vi "Duplicate.vi"(8 "error in":errorcluster, 10 "parameters":variant, 11 "node in":refnum<class "module editor node.lvclass">) -> (0 "error out":errorcluster, 3 "node copy out":refnum<class "module editor node.lvclass">)   [LabVIEW 2013, in "PL Framework Configuration Tool.lvlib" / "module editor node.lvclass"]
doc: "Implements the specific behavior of a node when it is being duplicated\nCan be used to change the name of the new node for example adding Copy to it. \nCopyright 2015 National Instruments Corporation\n\nLicensed under the Apache License, Version 2.0 (the \"License\"); you may not use this file except in compliance with the License. You may obtain a copy of the License at http://www.apache.org/licenses/LICENSE-2.0\nUnless required by applicable law or agreed to in writing, software distributed under the License is distributed on an \"AS IS\" BASIS, WITHOUT WARRANTIES OR CONDITIONS OF ANY KIND, either express or implied. See the License for the specific language governing permissions and limitations under the License."
uses:
  module editor node.lvclass
  TBM Configuration Node/TBM Configuration Node.lvclass
  <vilib>/NI/Configuration Framework/Node/NISE_CEF_Node.lvclass
  Targets/Targets.lvclass
  <vilib>/NI/Configuration Framework/serializable configuration/NISE_CEF_serializable configuration.lvclass
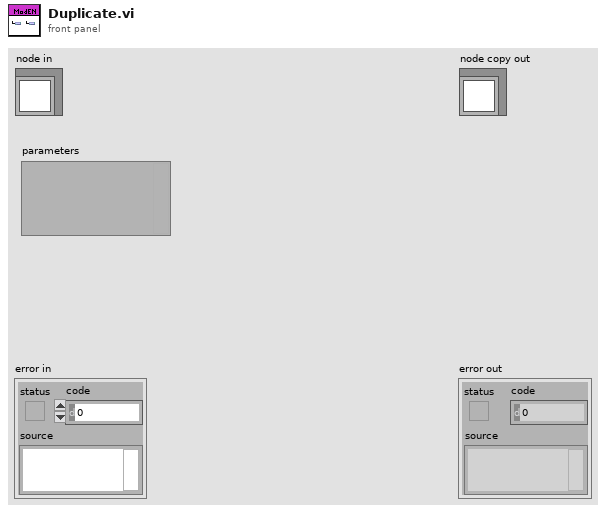
[diagram p1: front panel]
types:
  T1 = typedef "NISE_CEF_Node.lvclass/NodeRef.ctl" = refnum<data-value>
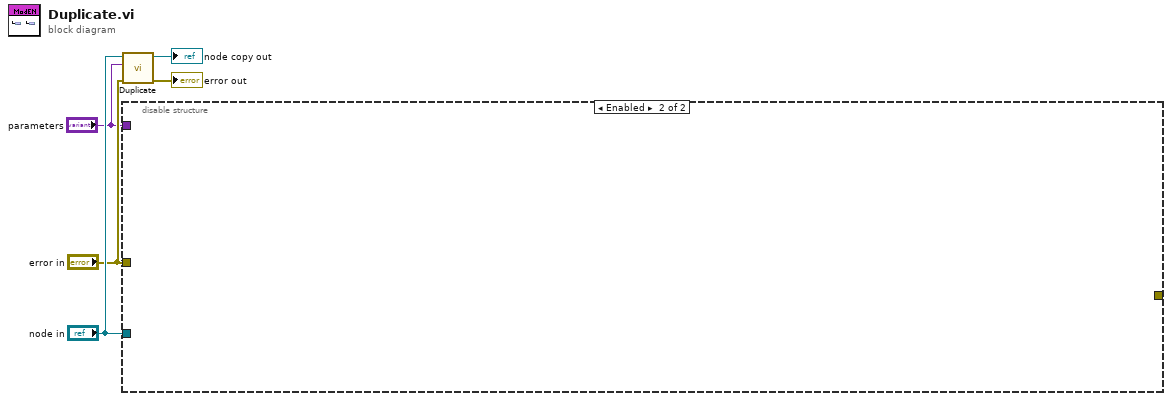
[diagram p0: block diagram]
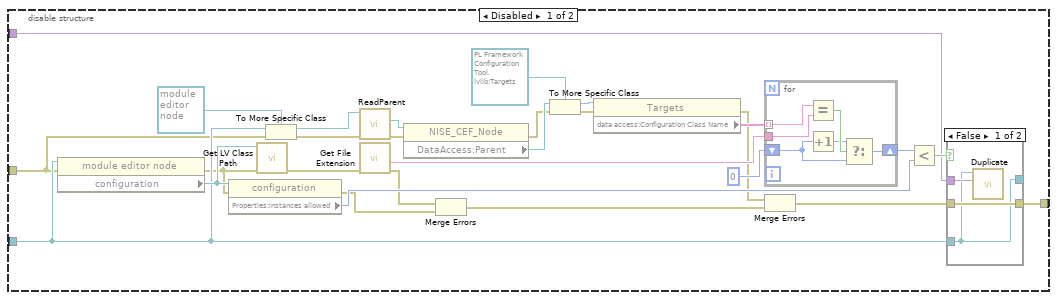
[diagram p2: hidden frame]
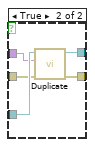
[diagram p3: hidden frame]
diagram:
  n1 = call-parent "Duplicate.vi"("error in"="error in", "parameters"="parameters", "node in"="node in") -> ("error out"=→"error out":errorcluster, "node copy out"=→"node copy out":refnum<class "module editor node.lvclass">)  [unwired: 7 in]
  n2 = disable-structure shown="Enabled" {
    disable-tunnel: "node in" -> [w19 _]
    disable-tunnel: [w18 _] -> _
    disable-tunnel: "error in" -> [w12 _]
    disable-tunnel: "parameters" -> [w6 _]
    frame Disabled {
      n3 = property class="module editor node"(reference=w19, error in=w12) -> (error out=w11:errorcluster, "configuration"=w25:refnum<class "NISE_CEF_serializable configuration.lvclass">)  [unwired: 1 out]
      n4 = property class="configuration"(reference=w25, error in=w11) -> (error out=w9:errorcluster, "Properties:instances allowed"=w21:i32)  [unwired: 1 out]
      n5 = call <vilib>:"Get LV Class Path.vi"("error in (no error)"=w11, "object"=w25) -> ("error out"=w27:errorcluster)  [unwired: 8 in, 1 out]
      n6 = To More Specific Class(target class=refnum<class "module editor node.lvclass"> refnum ("Tag Editor Core:module editor node"), reference=w19, error in=w12) -> (specific class reference=w32:refnum<class "module editor node.lvclass">, error out=w8:errorcluster)
      n7 = call <vilib>:"ReadParent.vi"("error in"=w8, "node in"=w32) -> ("error out"=w7:errorcluster, "parent"=w31:T1)  [unwired: 7 in, 1 out]
      n8 = call <vilib>:"Get File Extension.vi"("error in (no error)"=w27) -> ("error out"=w13:errorcluster, "filename without extension"=w24:string)  [unwired: 7 in, 2 out]
      n9 = property class="NISE_CEF_Node"(reference=w31, error in=w7) -> (error out=w16:errorcluster, "DataAccess:Parent"=w30:T1)  [unwired: 1 out]
      n10 = Merge Errors(w13, w9) -> (w10:errorcluster)
      n11 = To More Specific Class(target class=refnum<data-value> refnum, reference=w30, error in=w16) -> (specific class reference=w28:refnum<data-value>, error out=w17:errorcluster)
      n12 = property class="Targets"(reference=w28, error in=w17) -> (error out=w14:errorcluster, "data access:Configuration Class Name"=w26:string[])  [unwired: 1 out]
      n13 = for {
        tunnel: w26 -> [w47] mode=indexing
        tunnel: w24 -> [w46]
        shift-right: [w42] -> w22
        shift-left: 0 -> [w44]
        n14 = Equal?(x=w47, y=w46) -> (x = y?=w45:bool)
        n15 = Increment(x=w44) -> (x+1=w43:i32)
        n16 = Select(t=w43, s=w45, f=w44) -> (s? t:f=w42:i32)
      }
      n17 = Merge Errors(w14, w10) -> (w15:errorcluster)
      n18 = Less?(x=w22, y=w21) -> (x < y?=w20:bool)
      n19 = case shown="False" w20 {
        tunnel: w19 -> [w34 w41]
        tunnel: [w34 w40] -> _
        tunnel: [w36 w39] -> w18
        tunnel: w15 -> [w36 w38]
        tunnel: w6 -> [w35 w37]
        frame False {
          n20 = call-parent "Duplicate.vi"("parameters"=w35, "node in"=w34) -> ()  [unwired: 8 in, 2 out]
        }
        frame True {
          n21 = call-parent "Duplicate.vi"("error in"=w38, "parameters"=w37, "node in"=w41) -> ("error out"=w39:errorcluster, "node copy out"=w40:refnum<class "module editor node.lvclass">)  [unwired: 7 in]
        }
      }
    }
    frame Enabled {
    }
  }
